vi "source_check_compliance.vi"(10 "Target voltage":dbl, 11 "Actual voltage":dbl) -> (3 "Is compliance?":bool)   [LabVIEW 2020]
doc: "Determines if compliance is reached from difference in desired and actual voltage."
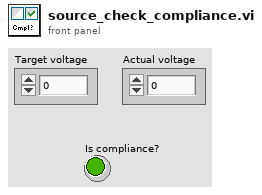
[diagram p1: front panel]
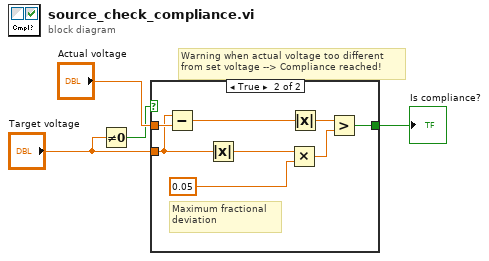
[diagram p0: block diagram]
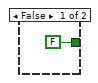
[diagram p2: hidden frame]
diagram:
  # "Warning when actual voltage too different\nfrom set voltage --> Compliance reached!"
  n1 = Not Equal To 0?(x="Target voltage") -> (x != 0?=w1:bool)
  n2 = case shown="True" w1 {
    tunnel: "Actual voltage" -> [_ w9]
    tunnel: [FALSE w8] -> w3
    tunnel: "Target voltage" -> [_ w6]
    frame False {
    }
    frame True {
      # "Maximum fractional\ndeviation"
      n3 = Subtract(x=w6, y=w9) -> (x-y=w13:dbl)
      n4 = Absolute Value(x=w6) -> (abs(x)=w7:dbl)
      n5 = Multiply(x=w7, y=0.05) -> (x*y=w11:dbl)
      n6 = Absolute Value(x=w13) -> (abs(x)=w12:dbl)
      n7 = Greater?(x=w12, y=w11) -> (0:w8:bool)
    }
  }
  "Is compliance?" <- w3
